vi "Baum Welch Single Iteration.vi"(10 "Observed states":i32[](array[numeric]), 11 "Init HMM":T1) -> (2 "Log10(Prob)":dbl, 3 "Estimated HMM":T1)   [LabVIEW 2014, in "HMM.lvlib"]
uses:
  HMM.lvlib
  Control/HMM Cluster.ctl
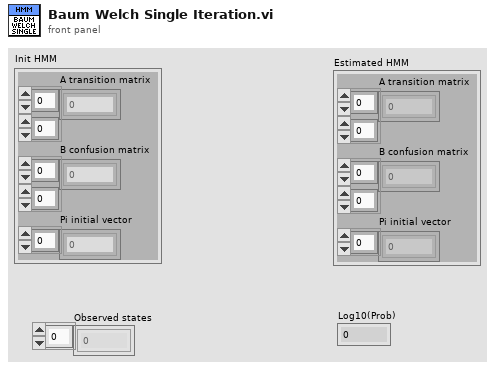
[diagram p1: front panel]
types:
  T1 = typedef "HMM.lvlib/HMM Cluster.ctl" = cluster{"A transition matrix":dbl[][], "B confusion matrix":dbl[][], "Pi initial vector":dbl[]}
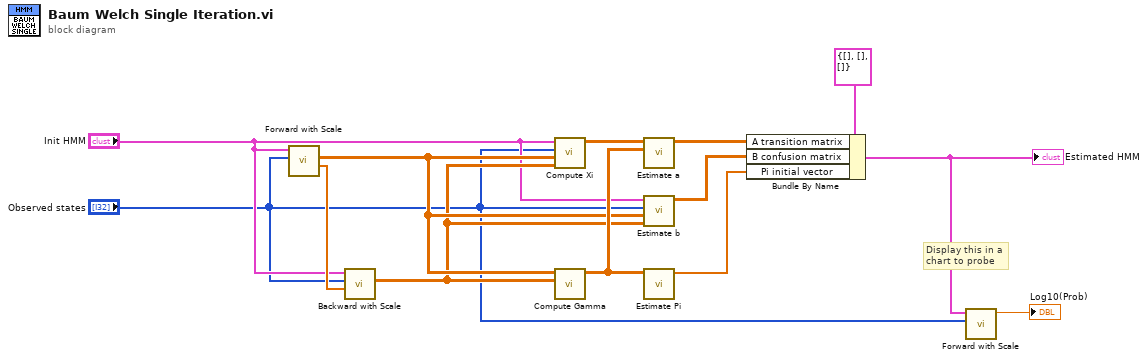
[diagram p0: block diagram]
diagram:
  # "Display this in a\nchart to probe"
  n1 = call "Forward with Scale.vi"("O Observed Sequence"="Observed states", "HMM Cluster"="Init HMM") -> ("Scale factor"=w7:dbl[], "Scaled Alpha"=w6:dbl[][])  [unwired: 6 in, 2 out]
  n2 = call "Backward with Scale.vi"("Scale factor"=w7, "O Observed Sequence"="Observed states", "HMM Cluster"="Init HMM") -> ("Beta Partial Probalility"=w5:dbl[][])  [unwired: 8 in]
  n3 = call "Compute Xi.vi"("Beta"=w5, "Alpha"=w6, "Observed sequence O"="Observed states", "HMM Cluster"="Init HMM") -> ("Xi"=w13:dbl[][][])  [unwired: 7 in]
  n4 = call "Compute Gamma.vi"("Beta"=w5, "Alpha"=w6) -> ("Gamma"=w11:dbl[][])  [unwired: 9 in]
  n5 = call "Estimate a.vi"("Gamma"=w11, "Xi"=w13) -> ("Estimated a"=w9:dbl[][])  [unwired: 9 in]
  n6 = call "Estimate b.vi"("Beta"=w5, "Alpha"=w6, "Observed states"="Observed states", "HMM Cluster"="Init HMM") -> ("Estimated b"=w10:dbl[][])  [unwired: 7 in]
  n7 = call "Estimate Pi.vi"("Gamma"=w11) -> ("Estimated Pi"=w12:dbl[])  [unwired: 10 in]
  n8 = Bundle By Name(cluster=T1 {"A transition matrix"=[], "B confusion matrix"=[], "Pi initial vector"=[]} ("HMM Cluster"), "A transition matrix"=w9, "B confusion matrix"=w10, "Pi initial vector"=w12) -> (w8:T1)
  "Estimated HMM" <- w8
  n9 = call "Forward with Scale.vi"("O Observed Sequence"="Observed states", "HMM Cluster"=w8) -> ("Log10(Prob)"=→"Log10(Prob)":dbl)  [unwired: 6 in, 3 out]
